vi "ArmFF_MaxAchieveAccel.vi"(8 "Velocity":dbl, 9 "Angle":dbl, 10 "MaxVoltage":dbl, 11 "in ARM_FF":T1 {"kCos" format="%13.5p"; "Ka" format="%13.5p"; "Kv" format="%13.5p"; "Ks" format="%13.5p"}) -> (3 "MaxAccel":dbl)   [LabVIEW 2019, in "Trajectory_Library.lvlib"]
doc: "Calculates the maximum achievable acceleration given a maximum voltage supply, a position, and a velocity. Useful for ensuring that velocity and acceleration constraints for a trapezoidal profile are simultaneously achievable - enter the velocity constraint, and this will give you a simultaneously-achievable acceleration constraint.\n \nInputs: \n - ArmFF -- The ArmFF data cluster\n - maxVoltage -- The maximum voltage that can be supplied to the arm.\n - angle -- The angle of the arm.\n - velocity -- The velocity of the arm.\n\nOutputs:\n - MaxAccel -- The maximum possible acceleration at the given velocity."
uses:
  Trajectory_Library.lvlib
  TypeDef/ARM_FF.ctl
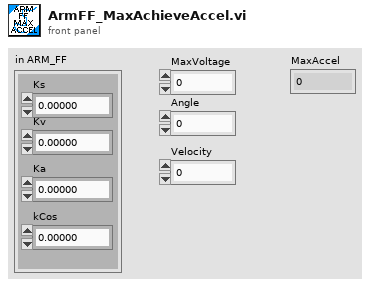
[diagram p1: front panel]
types:
  T1 = typedef "Trajectory_Library.lvlib/ARM_FF.ctl" = cluster{"Ks":dbl, "Kv":dbl, "Ka":dbl, "kCos":dbl}
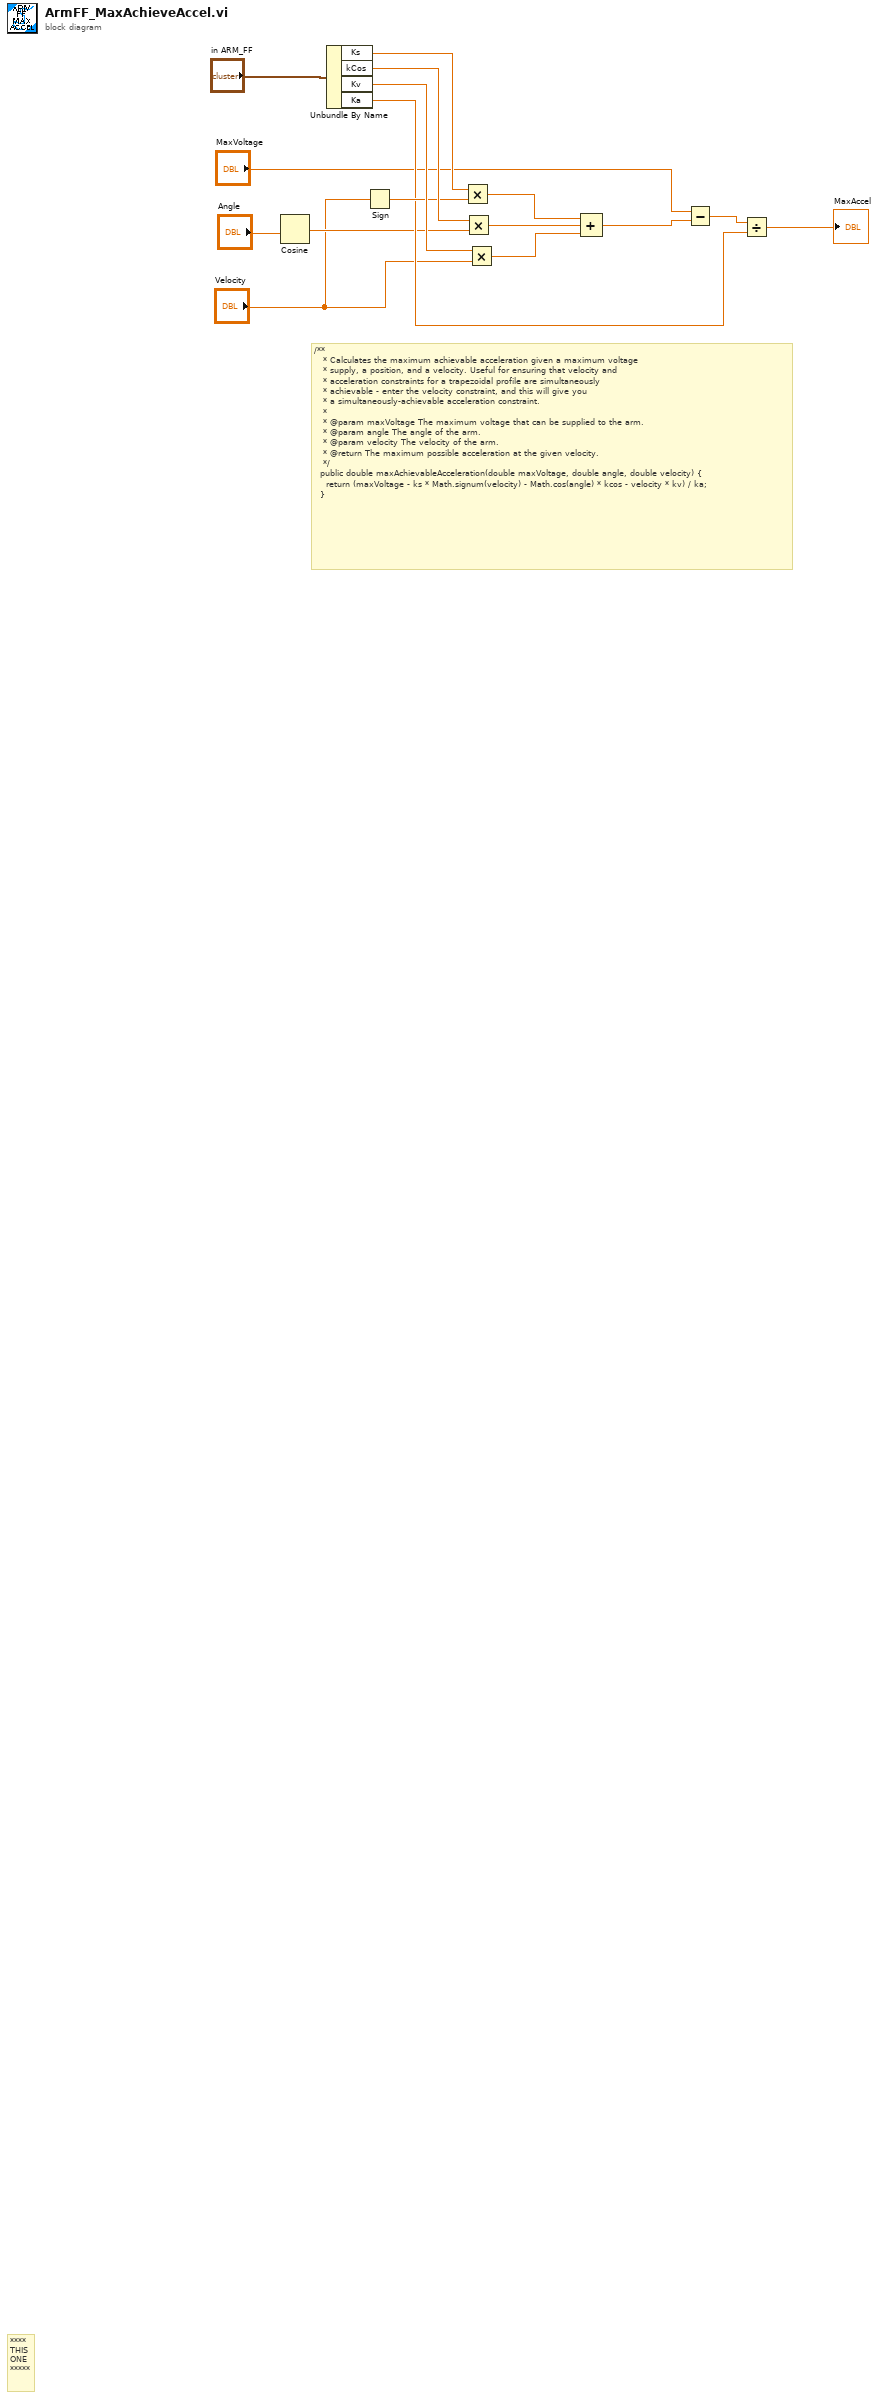
[diagram p0: block diagram]
diagram:
  # "/**\n   * Calculates the maximum achievable acceleration given a maximum voltage\n   * supply, a position, and a velocity. Useful for ensuring that velocity and\n   * acceleration constraints for a trapezoidal profile are simultaneously\n   * achievable - enter the velocity constraint, and this will give you\n   * a simultaneously-achievable acceleration constraint.\n   *\n   * @param maxVoltage The maximum voltage that can be supplied to the arm.\n   * @param angle The angle of the arm.\n   * @param velocity The velocity of the arm.\n   * @return The maximum possible acceleration at the given velocity.\n   */\n  public double maxAchievableAcceleration(double maxVoltage, double angle, double velocity) {\n    return (maxVoltage - ks * Math.signum(velocity) - Math.cos(angle) * kcos - velocity * kv) / ka;\n  }"
  # "****\nTHIS\nONE\n*****"
  n1 = Cosine(x="Angle") -> (cos(x)=w2:dbl)
  n2 = Unbundle By Name("in ARM_FF") -> ("Ks"=w12:dbl, "kCos"=w11:dbl, "Kv"=w10:dbl, "Ka"=w5:dbl)
  n3 = Sign(1:"Velocity") -> (0:w9:dbl)
  n4 = Multiply(x=w12, y=w9) -> (x*y=w15:dbl)
  n5 = Multiply(x=w11, y=w2) -> (x*y=w14:dbl)
  n6 = Multiply(x=w10, y="Velocity") -> (x*y=w13:dbl)
  n7 = Compound Arithmetic op=ADD(w15, w14, w13) -> (w8:dbl)
  n8 = Subtract(x="MaxVoltage", y=w8) -> (x-y=w7:dbl)
  n9 = Divide(x=w7, y=w5) -> (x/y=→"MaxAccel":dbl)
